vi "Fpga reg.vi"(8 "Mode":enum16{"Get", "Set"}(ring), 10 "FPGA VI Reference Set":refnum<k20>) -> (2 "FPGA VI Reference Out":refnum<k20>)   [LabVIEW 2019, in "my FPGA lib.lvlib"]
uses:
  my FPGA lib.lvlib
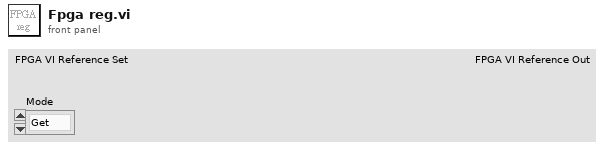
[diagram p1: front panel]
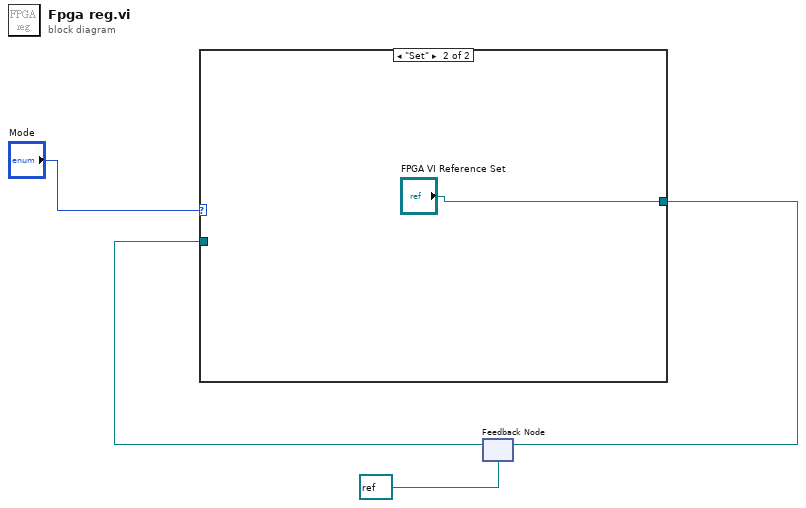
[diagram p0: block diagram]
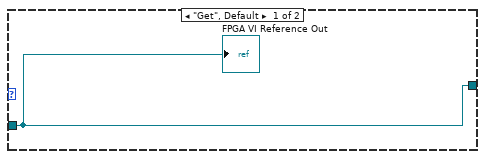
[diagram p2: hidden frame]
diagram:
  n1 = feedback #1(refnum<k20> refnum ("FPGA VI Reference Set")) -> (w2:refnum<k20>)
  n2 = case shown="\"Set\"" "Mode" {
    tunnel: [w5 "FPGA VI Reference Set"] -> w3
    tunnel: w2 -> [w5 _]
    frame "Get", Default {
      "FPGA VI Reference Out" <- w5
    }
    frame "Set" {
    }
  }
  n3 = feedback-in #1(w3) -> ()
